vi "Get Error.vi"(7 "scope":T2, 8 "error in (no error)":errorcluster, 10 "owner error":T3, 11 "error list <top>":variant) -> (0 "error out":errorcluster, 1 "attributes":string[](array[string]), 2 "error":T1, 3 "error list <top> dup":variant, 4 "found?":bool)   [LabVIEW 2017]
uses:
  Error Owner and ID.ctl
  Scope.ctl
  Error File Management/Controls/NI Error.ctl
  Error File Management/Error File Management.lvlib
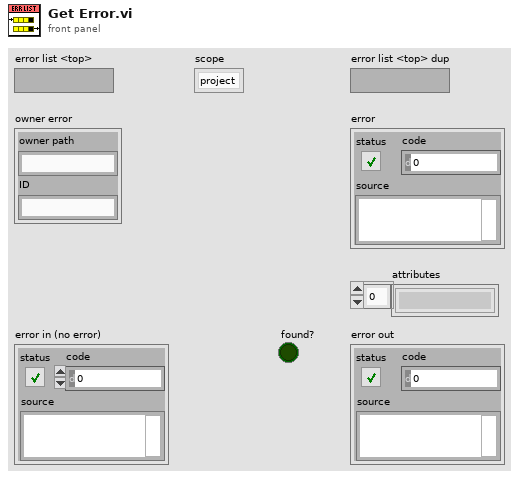
[diagram p1: front panel]
types:
  T1 = typedef "Error File Management.lvlib/NI Error.ctl" = errorcluster
  T2 = typedef "Scope.ctl" = enum16{"project", "global"}
  T3 = typedef "Error Owner and ID.ctl" = cluster{"owner path":string, "ID":string}
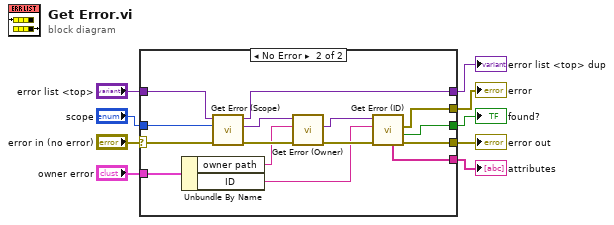
[diagram p0: block diagram]
diagram:
  n1 = case shown="No Error" "error in (no error)" {
    selector: "error in (no error)" -> [w11 w17]
    tunnel: "owner error" -> [_ w24]
    tunnel: "scope" -> [_ w19]
    tunnel: [w11 w18] -> w6
    tunnel: "error list <top>" -> [w10 w16]
    tunnel: [_ w15] -> w4
    tunnel: [_ w13] -> w3
    tunnel: [_ w14] -> w2
    tunnel: [w10 w12] -> w1
    frame Error {
    }
    frame No Error {
      n2 = Unbundle By Name(w24) -> ("owner path"=w22:string, "ID"=w23:string)
      n3 = call "Get Error (Scope).vi"("error in (no error)"=w17, "scope"=w19, "error list <top>"=w16) -> ("error out"=w25:errorcluster, "error list <scope>"=w20:variant, "error list <top> dup"=w12:variant)  [unwired: 5 in, 1 out]
      n4 = call "Get Error (Owner).vi"("error in (no error)"=w25, "owner"=w22, "error list <scope>"=w20) -> ("error out"=w26:errorcluster, "error list <owner>"=w21:variant)  [unwired: 5 in, 2 out]
      n5 = call "Get Error (ID).vi"("error in (no error)"=w26, "ID"=w23, "error list <owner>"=w21) -> ("error out"=w18:errorcluster, "found?"=w14:bool, "error"=w15:T1, "attributes"=w13:string[])  [unwired: 4 in, 1 out]
    }
  }
  "error out" <- w6
  "error" <- w4
  "attributes" <- w3
  "found?" <- w2
  "error list <top> dup" <- w1
